vi "GetCurrentPosition.vi"(8 "Error In":errorcluster) -> (0 "Error Out":errorcluster, 1 "Z":dbl, 2 "Y":dbl, 3 "X":dbl)   [LabVIEW 2012]
doc: "SciScan 1.2 160622"
uses:
  GFG/GFGnumericGet.vi
  GFG/GFG library.lvlib
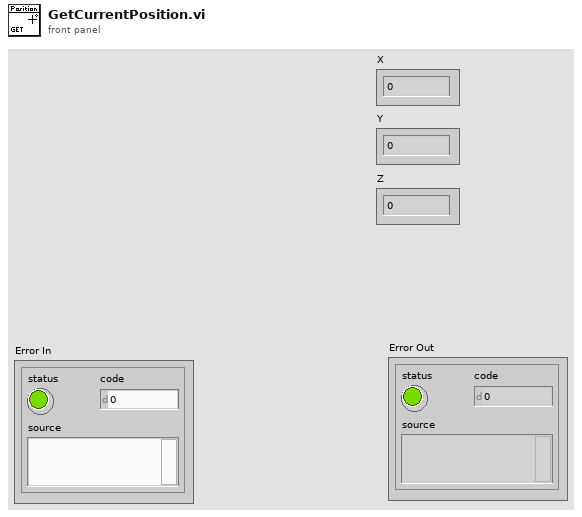
[diagram p1: front panel]
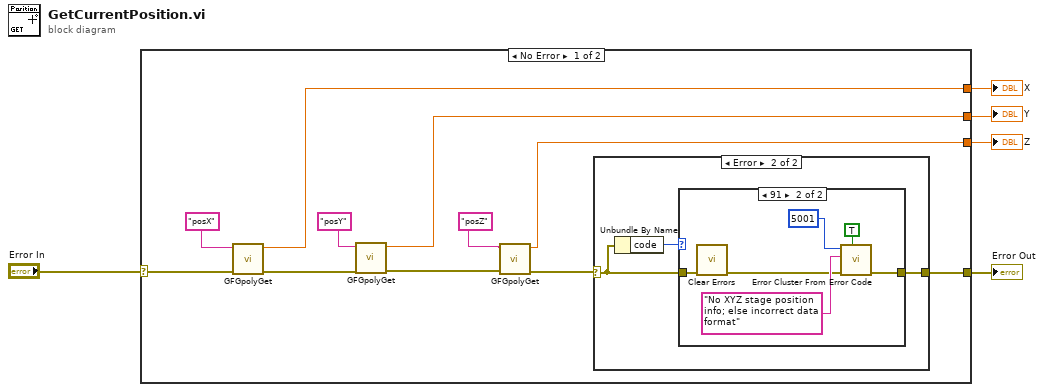
[diagram p0: block diagram]
diagram:
  n1 = case shown="No Error" "Error In" {
    selector: "Error In" -> [w15 w28]
    tunnel: [w16 w28] -> w4
    tunnel: [w13 _] -> w3
    tunnel: [w9 _] -> w2
    tunnel: [w7 _] -> w1
    frame No Error {
      n2 = call-poly "GFGpolyGet.vi"("error in (no error)"=w15, "Variable Name in"="posX") -> ("error out"=w11:errorcluster, "Numeric"=w13:dbl)  [unwired: 7 in, 1 out]
      n3 = call-poly "GFGpolyGet.vi"("error in (no error)"=w11, "Variable Name in"="posY") -> ("error out"=w10:errorcluster, "Numeric"=w9:dbl)  [unwired: 7 in, 1 out]
      n4 = call-poly "GFGpolyGet.vi"("error in (no error)"=w10, "Variable Name in"="posZ") -> ("error out"=w6:errorcluster, "Numeric"=w7:dbl)  [unwired: 7 in, 1 out]
      n5 = case shown="Error" w6 {
        selector: w6 -> [w17 w19]
        tunnel: [w17 w18] -> w16
        frame No Error {
        }
        frame Error {
          n6 = Unbundle By Name(w19) -> ("code"=w20:i32)
          n7 = case shown="91" w20 {
            tunnel: w19 -> [w21 w27]
            tunnel: [w21 w23] -> w18
            frame 0, Default {
            }
            frame 91 {
              n8 = call <vilib>:"Clear Errors.vi"("error in (no error)"=w27) -> ("error out"=w24:errorcluster)  [unwired: 6 in]
              n9 = call <vilib>:"Error Cluster From Error Code.vi"("show call chain? (False)"=TRUE, "error in (no error)"=w24, "error message (\"\")"="No XYZ stage position  info; else incorrect data format" ("error message (\"\")"), "error code (0)"=5001) -> ("error out"=w23:errorcluster)  [unwired: 5 in]
            }
          }
        }
      }
    }
    frame Error {
    }
  }
  "Error Out" <- w4
  "X" <- w3
  "Y" <- w2
  "Z" <- w1
